vi "myComplemetary Filter.vi"() -> ()   [LabVIEW 2011]
doc: "I. Description:\nThis example demonstrates how to output a single Voltage Update (Sample) to an Analog Output Channel.\n\nII. Instructions for Running:\n1. Select the Physical Channel to correspond to where your signal is output on the DAQ device.\n2. Enter the Minimum and Maximum Voltage Ranges\nNote: Use the Acq One Sample example to verify you are generating the correct output on the DAQ device\n\nIII. Block Diagram Steps:\n1. Create an Analog Output Voltage Channel\n2. Use the Write VI to Output 1 Sample to 1 Channel on the Data\nAcquisition Card. \n3. Call the Clear Task VI to clear the Task.\n4. Use the popup dialog box to display an error if any. \n\nIV. I/O Connections Overview:\nMake sure your signal output terminal matches the Physical Channel I/O Control. For further connection information, refer to your hardware reference manual."
uses:
  <vilib>/DAQmx/read.llb/DAQmx Read (Analog 1D DBL NChan 1Samp).vi
  <vilib>/DAQmx/create/channels.llb/DAQmx Create Channel (AI-Voltage-Basic).vi
  <vilib>/DAQmx/miscellaneous.llb/DAQmx Fill In Error Info.vi
  <vilib>/picture/3D Picture Control/NI_3D Picture Control.lvlib
panel:
  out "Data Display":T1(graph)
  in  "Filter Coefficient a":dbl(slide)=0.7473684210526316 scale=0.0..1.0
  in  "Stop":bool
  in  "Initialize Accel":bool
  in  "Initialize Gyro":bool
  in  "Sensitivity (mV/g)":dbl=330.0
  in  "Sensitivity (mV/°/s)":dbl=8.3
  out "Time Constant (s)":dbl
  out "Gyro":refnum<vi>(3d-picture)
  out "Accelerometer":refnum<vi>(3d-picture)
  in  "physical channels":tag="myDAQ1/ai0:1"
  out "Filtered Accelerometer & Gyro":refnum<vi>(3d-picture)
  # "myComplementary Filter"
  # "Chart Information"
  # "Channel Parameters"
  # "Gyro Parameters"
  # "Accelerometer Parameters"
  # "Complementary Filter Parameters"
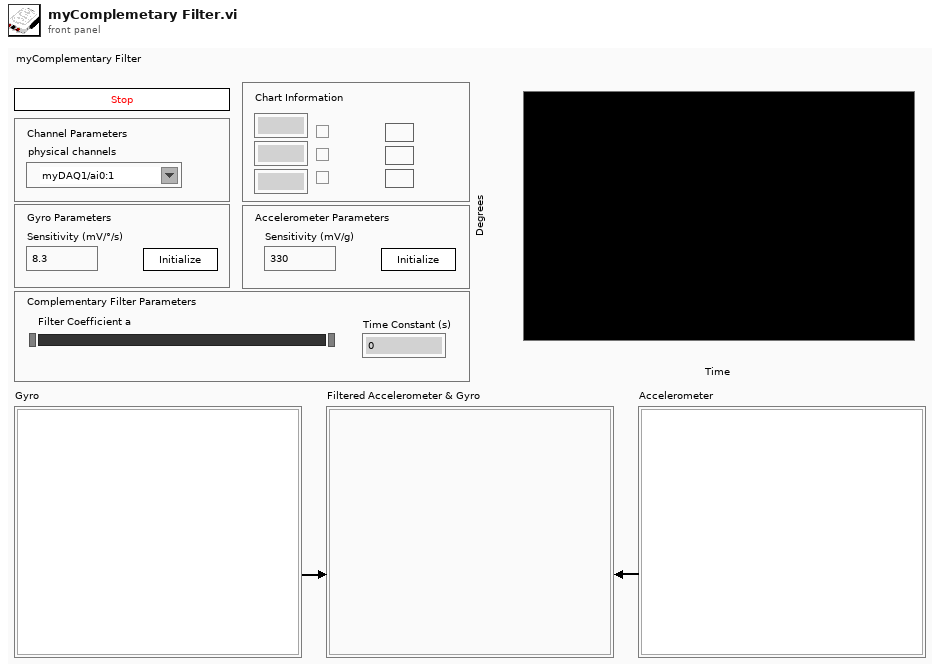
[diagram p1: front panel]
types:
  T1 = cluster{"Rate of turn (°/s)":dbl, "Angle from horizontal (°)":dbl, "Filtered":dbl}
  T2 = cluster{"Red":sgl, "Green":sgl, "Blue":sgl, "Alpha":sgl}
  T3 = cluster{"Degrees":dbl, "Angle from horizontal (°)":dbl, "Filtered":dbl}
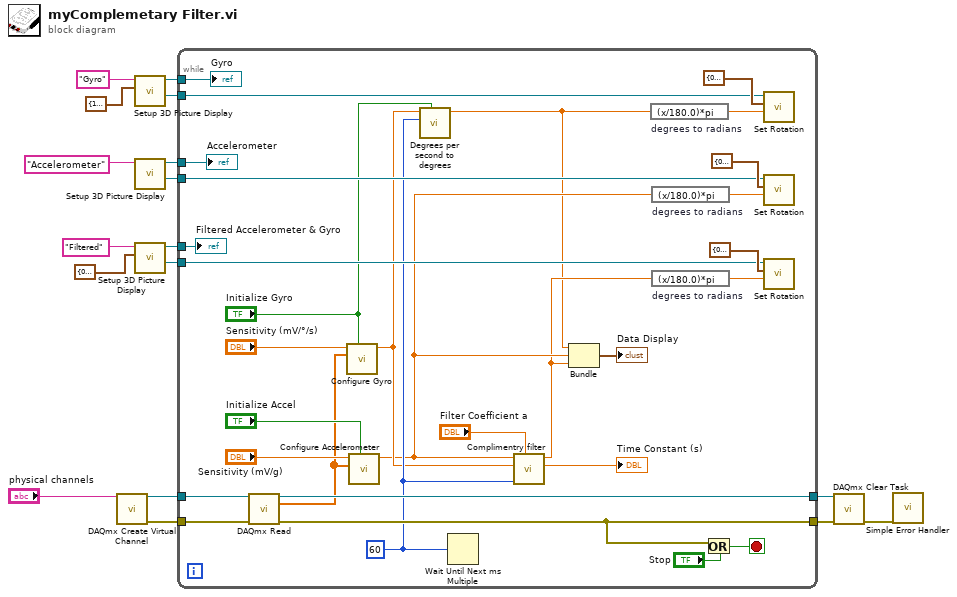
[diagram p0: block diagram]
diagram:
  n1 = call-poly <vilib>:"DAQmx Create Virtual Channel.vi"("physical channels"="physical channels") -> ("task out"=w13:refnum<k21>, "error out"=w12:errorcluster)  [unwired: 13 in]
  n2 = call "Setup 3D Picture Display.vi"("Color"=T2 {"Red"=1.0, "Green"=1.0, "Blue"=1.0, "Alpha"=1.0}, "Name"="Gyro") -> ("SceneObject out"=w11:refnum<vi>, "Scene:New Object"=w10:refnum<vi>)  [unwired: 8 in]
  n3 = call "Setup 3D Picture Display.vi"("Name"="Accelerometer") -> ("SceneObject out"=w7:refnum<vi>, "Scene:New Object"=w8:refnum<vi>)  [unwired: 9 in]
  n4 = call "Setup 3D Picture Display.vi"("Color"=T2 {"Red"=0.0, "Green"=1.0, "Blue"=0.0, "Alpha"=1.0}, "Name"="Filtered") -> ("SceneObject out"=w4:refnum<vi>, "Scene:New Object"=w5:refnum<vi>)  [unwired: 8 in]
  n5 = while {
    tunnel: [w46] -> w16
    tunnel: [w48] -> w15
    tunnel: w13 -> [w45]
    tunnel: w12 -> [w44]
    tunnel: w5 -> [w43]
    tunnel: w4 -> [w40]
    tunnel: w8 -> [w39]
    tunnel: w7 -> [w36]
    tunnel: w11 -> [w31]
    tunnel: w10 -> [w30]
    stop <- w47 stop-if-true
    w24 = u32 60 ("millisecond multiple")
    n6 = call-poly <vilib>:"DAQmx Read.vi"("task/channels in"=w45, "error in"=w44) -> ("task out"=w48:refnum<k21>, "data"=w26:dbl[], "error out"=w46:errorcluster)  [unwired: 11 in]
    n7 = call "Configure Gyro.vi"("Initialize"="Initialize Gyro", "data"=w26, "Sensitivity (mV/°/s)"="Sensitivity (mV/°/s)") -> ("Rate of turn (°/s)"=w22:dbl)  [unwired: 8 in]
    n8 = call "Configure Accelerometer.vi"("Initialize"="Initialize Accel", "data"=w26, "Sensitivity (mV/g)"="Sensitivity (mV/g)") -> ("Angle from horizontal (°)"=w21:dbl)  [unwired: 8 in]
    n9 = call "Degrees per second to degrees.vi"("Initialize"="Initialize Gyro", "Sample time (ms)"=w24, "Rate of turn (°/s)"=w22) -> ("Degrees"=w18:dbl)  [unwired: 8 in]
    n10 = Wait Until Next ms Multiple(millisecond multiple=w24) -> ()  [unwired: 1 out]
    n11 = call "Complimentry filter.vi"("Filter Coefficient a"="Filter Coefficient a", "dt (ms)"=w24, "Gyro (degrees/second)"=w22, "Accelerometer (degrees)"=w21) -> ("timeConstant"=→"Time Constant (s)":dbl, "Filtered"=w20:dbl)  [unwired: 6 in]
    n12 = Bundle("Degrees"=w18, "Angle from horizontal (°)"=w21, "Filtered"=w20) -> (→"Data Display":T3)  [unwired: 1 in]
    n13 = expression code="(x/180.0)*pi" "degrees to radians"(w18) -> (w34:dbl)
    n14 = expression code="(x/180.0)*pi" "degrees to radians"(w21) -> (w38:dbl)
    n15 = expression code="(x/180.0)*pi" "degrees to radians"(w20) -> (w41:dbl)
    n16 = Or(x=w46, y="Stop") -> (x .or. y?=w47:bool)
    n17 = call <vilib>:"Set Rotation.vi"("Angle"=w34, "Axis"=cluster{"X":sgl, "Y":sgl, "Z":sgl} {"X"=0.0, "Y"=1.0, "Z"=0.0}, "Scene Object"=w31) -> ()  [unwired: 7 in, 2 out]
    n18 = call <vilib>:"Set Rotation.vi"("Angle"=w38, "Axis"=cluster{"X":sgl, "Y":sgl, "Z":sgl} {"X"=0.0, "Y"=1.0, "Z"=0.0}, "Scene Object"=w36) -> ()  [unwired: 7 in, 2 out]
    n19 = call <vilib>:"Set Rotation.vi"("Angle"=w41, "Axis"=cluster{"X":sgl, "Y":sgl, "Z":sgl} {"X"=0.0, "Y"=1.0, "Z"=0.0}, "Scene Object"=w40) -> ()  [unwired: 7 in, 2 out]
    "Filtered Accelerometer & Gyro" <- w43
    "Accelerometer" <- w39
    "Gyro" <- w30
  }
  n20 = call <vilib>:"DAQmx Clear Task.vi"("task in"=w15, "error in"=w16) -> ("error out"=w14:errorcluster)  [unwired: 13 in]
  n21 = call <vilib>:"Simple Error Handler.vi"("error in (no error)"=w14) -> ()  [unwired: 4 in, 5 out]
